vi "Read Data.vi"(8 "error in (no error)":errorcluster, 11 "Dbl Array in":refnum<class "Dbl Array.lvclass">) -> (0 "error out":errorcluster, 2 "Data":dbl[](array[numeric]), 3 "Dbl Array out":refnum<class "Dbl Array.lvclass">)   [LabVIEW 2018, in "Base Data Class.lvlib" / "Dbl Array.lvclass"]
uses:
  Dbl Array.lvclass
  Dbl Array.lvclass/Dbl Array.ctl
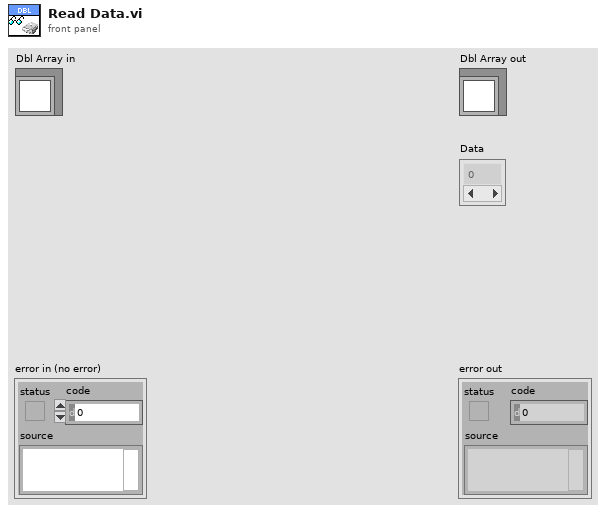
[diagram p1: front panel]
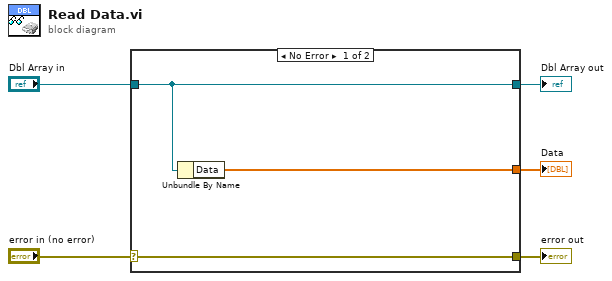
[diagram p0: block diagram]
diagram:
  n1 = case shown="No Error" "error in (no error)" {
    selector: "error in (no error)" -> [w8 w9]
    tunnel: [w8 w9] -> w4
    tunnel: [w7 w10] -> w2
    tunnel: "Dbl Array in" -> [w7 w10]
    tunnel: [w6 _] -> w1
    frame No Error {
      n2 = Unbundle By Name(w7) -> ("Data"=w6:dbl[])
    }
    frame Error {
    }
  }
  "error out" <- w4
  "Dbl Array out" <- w2
  "Data" <- w1
